vi "OpenCVCam_GetPicture.vi"(8 "error in (no error)":errorcluster, 10 "Cmd Data":variant, 11 "OpenCVCam in":refnum<class>) -> (0 "error out":errorcluster, 2 "Reply Data":variant, 3 "OpenCVCam out":refnum<class>, 4 "Exit":bool)   [LabVIEW 2021, in "OpenCVCam.lvclass"]
uses:
  OpenCVCam.lvclass
  OpenCVCam_UiCallBackEvents.ctl
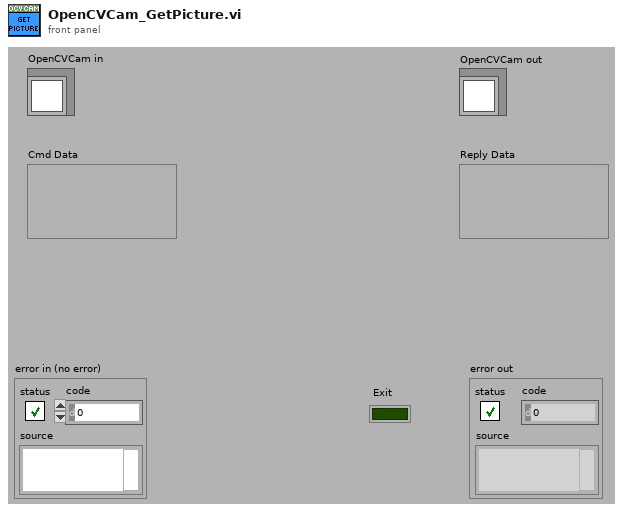
[diagram p1: front panel]
types:
  T1 = typedef "OpenCVCam.lvclass/OpenCVCam_UiCallBackEvents.ctl" = enum16{"Default", "PersistentDataUpdated", "NewPicture", "Worker 1: Do Something"}
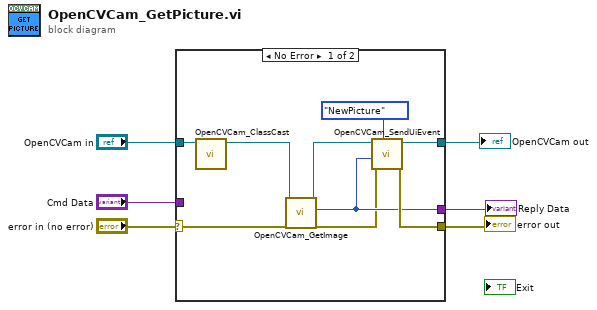
[diagram p0: block diagram]
diagram:
  n1 = case shown="No Error" "error in (no error)" {
    selector: "error in (no error)" -> [w13 w18]
    tunnel: [w11 w18] -> w5
    tunnel: [w10 w17] -> w3
    tunnel: "Cmd Data" -> [_ w17]
    tunnel: "OpenCVCam in" -> [w15 w16]
    tunnel: [w12 w16] -> w1
    frame No Error {
      n2 = call "OpenCVCam_ClassCast.vi"("OpenCVCam in"=w15) -> ("OpenCVCam out"=w14:refnum<class "OpenCVCam.lvclass">)  [unwired: 10 in]
      n3 = call "OpenCVCam_GetImage.vi"("error in (no error)"=w13, "OpenCVCam in"=w14) -> ("error out"=w7:errorcluster, "new picture"=w10:picture, "OpenCVCam out"=w8:refnum<class "OpenCVCam.lvclass">)  [unwired: 7 in]
      n4 = call "OpenCVCam_SendUiEvent.vi"("UiEventNames"=OpenCVCam_UiCallBackEvents."NewPicture", "ErrorIn"=w7, "Data"=w10, "OpenCVCam in"=w8) -> ("ErrorOut"=w11:errorcluster, "OpenCVCam out"=w12:refnum<class "OpenCVCam.lvclass">)  [unwired: 6 in]
    }
    frame Error {
    }
  }
  "error out" <- w5
  "OpenCVCam out" <- w1
  "Reply Data" <- w3
